vi "ptbypt derivatives (SubVI).vi"(11 "Array of Double":dbl[](array[numeric])) -> (1 "outer cmd [deg]":T1, 2 "middle cmd [deg]":T2, 3 "inner cmd [deg]":T1)   [LabVIEW 2017]
uses:
  <vilib>/ptbypt/NI_PtbyPt.lvlib
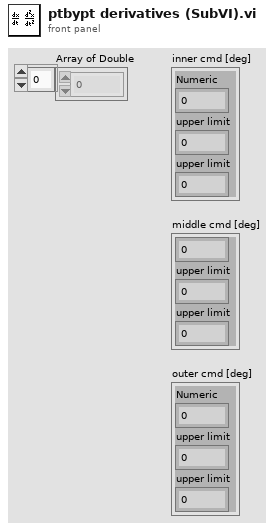
[diagram p1: front panel]
types:
  T1 = cluster{"Numeric":dbl, "upper limit":dbl, "upper limit":dbl}
  T2 = cluster{dbl, "upper limit":dbl, "upper limit":dbl}
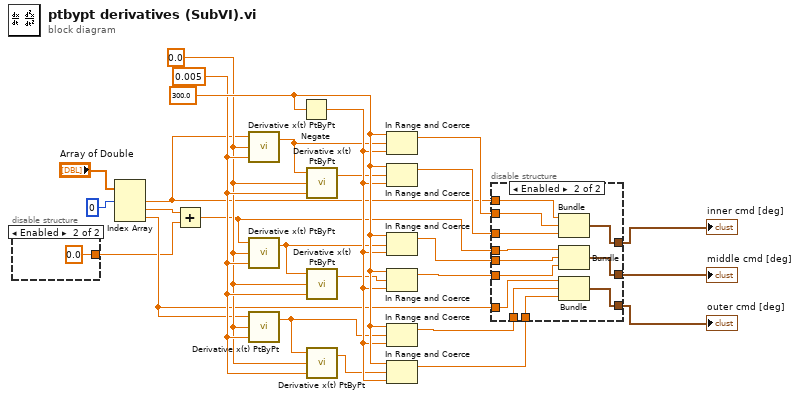
[diagram p0: block diagram]
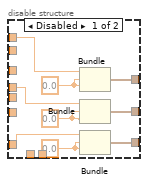
[diagram p2: hidden frame]
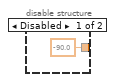
[diagram p3: hidden frame]
diagram:
  w26 = 300.0 ("upper limit")
  w11 = 0.0 ("initial condition")
  w12 = 0.005 ("dt")
  n1 = disable-structure shown="Enabled" {
    disable-tunnel: [-90.0 ("y") 0.0 ("y")] -> w3
    frame Disabled {
    }
    frame Enabled {
    }
  }
  n2 = Index Array(array="Array of Double", index #1=0 ("index")) -> (element #1=w8:dbl, element #2=w4:dbl, element #3=w10:dbl)  [unwired: 2 in]
  n3 = Add(x=w4, y=w3) -> (x+y=w9:dbl)
  n4 = call <vilib>:"Derivative x(t) PtByPt.vi"("dt"=w12, "initial condition"=w11, "x"=w8) -> ("dx/dt"=w19:dbl)  [unwired: 1 in, 1 out]
  n5 = call <vilib>:"Derivative x(t) PtByPt.vi"("dt"=w12, "initial condition"=w11, "x"=w9) -> ("dx/dt"=w23:dbl)  [unwired: 1 in, 1 out]
  n6 = call <vilib>:"Derivative x(t) PtByPt.vi"("dt"=w12, "initial condition"=w11, "x"=w10) -> ("dx/dt"=w22:dbl)  [unwired: 1 in, 1 out]
  n7 = Negate(x=w26) -> (-x=w25:dbl)
  n8 = call <vilib>:"Derivative x(t) PtByPt.vi"("dt"=w12, "initial condition"=w11, "x"=w19) -> ("dx/dt"=w17:dbl)  [unwired: 1 in, 1 out]
  n9 = call <vilib>:"Derivative x(t) PtByPt.vi"("dt"=w12, "initial condition"=w11, "x"=w23) -> ("dx/dt"=w15:dbl)  [unwired: 1 in, 1 out]
  n10 = call <vilib>:"Derivative x(t) PtByPt.vi"("dt"=w12, "initial condition"=w11, "x"=w22) -> ("dx/dt"=w13:dbl)  [unwired: 1 in, 1 out]
  n11 = In Range and Coerce(upper limit=w26, x=w19, lower limit=w25) -> (coerced(x)=w20:dbl)  [unwired: 1 out]
  n12 = In Range and Coerce(upper limit=w26, x=w17, lower limit=w25) -> (coerced(x)=w18:dbl)  [unwired: 1 out]
  n13 = In Range and Coerce(upper limit=w26, x=w23, lower limit=w25) -> (coerced(x)=w24:dbl)  [unwired: 1 out]
  n14 = In Range and Coerce(upper limit=w26, x=w15, lower limit=w25) -> (coerced(x)=w16:dbl)  [unwired: 1 out]
  n15 = In Range and Coerce(upper limit=w26, x=w22, lower limit=w25) -> (coerced(x)=w21:dbl)  [unwired: 1 out]
  n16 = In Range and Coerce(upper limit=w26, x=w13, lower limit=w25) -> (coerced(x)=w14:dbl)  [unwired: 1 out]
  n17 = disable-structure shown="Enabled" {
    disable-tunnel: w9 -> [w37 w45]
    disable-tunnel: w10 -> [w36 w44]
    disable-tunnel: [w35 w49] -> w5
    disable-tunnel: [w34 w48] -> w6
    disable-tunnel: [w33 w47] -> w7
    disable-tunnel: w8 -> [w29 w46]
    disable-tunnel: w20 -> [_ w43]
    disable-tunnel: w18 -> [_ w42]
    disable-tunnel: w24 -> [_ w41]
    disable-tunnel: w16 -> [_ w40]
    disable-tunnel: w21 -> [_ w39]
    disable-tunnel: w14 -> [_ w38]
    frame Disabled {
      w32 = 0.0
      w31 = 0.0
      w30 = 0.0
      n18 = Bundle("Numeric"=w29, w31, w31) -> (w35:cluster{"Numeric":dbl, dbl, dbl})  [unwired: 1 in]
      n19 = Bundle(w37, w30, w30) -> (w34:cluster{dbl, dbl, dbl})  [unwired: 1 in]
      n20 = Bundle("Numeric"=w36, w32, w32) -> (w33:cluster{"Numeric":dbl, dbl, dbl})  [unwired: 1 in]
    }
    frame Enabled {
      n21 = Bundle("Numeric"=w46, "upper limit"=w43, "upper limit"=w42) -> (w49:T1)  [unwired: 1 in]
      n22 = Bundle(w45, "upper limit"=w41, "upper limit"=w40) -> (w48:T2)  [unwired: 1 in]
      n23 = Bundle("Numeric"=w44, "upper limit"=w39, "upper limit"=w38) -> (w47:T1)  [unwired: 1 in]
    }
  }
  "outer cmd [deg]" <- w7
  "middle cmd [deg]" <- w6
  "inner cmd [deg]" <- w5
